vi "FTW-Container-Value-String.vi"(0 "JSON":refnum<class "FTW-Container.lvclass">, 11 "error in":errorcluster) -> (4 "JSON out":refnum<class "FTW-Container.lvclass">, 8 "Value":string, 15 "error out":errorcluster)   [LabVIEW 2015, in "FTW-Container.lvclass"]
uses:
  FTW-Container.lvclass
  FTW-Container.lvclass/FTW-Container.ctl
  <vilib>/Utility/Data Type/NI_Data Type.lvlib
panel:
  # "Inputs"
  # "Outputs"
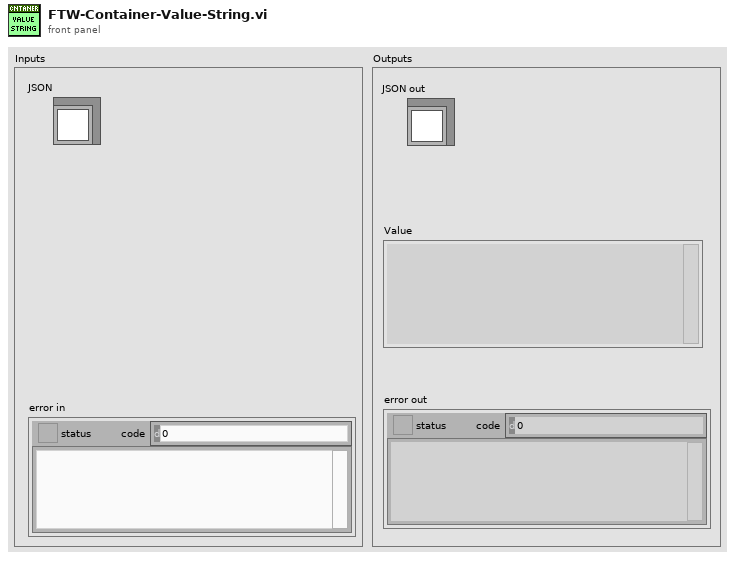
[diagram p1: front panel]
types:
  T1 = typedef "NI_Data Type.lvlib/Data Type.ctl" = enum8{"Invalid Type", "Void", "I8", "I16", "I32", "I64", "U8", "U16", "U32", "U64", "Single Float", "Double Float", "Extended Float", "Single Complex", "Double Complex", "Extended Complex", "Enum U8", "Enum U16", "Enum U32", "Enum U64", "Single Float With Unit", "Double Float With Unit", "Extended Float With Unit", "Single Complex with Unit", "Double Complex with Unit", "Extended Complex with Unit", "Boolean", "String", "Path", "Picture", "Tag", "Array", "Cluster", "Variant", "LV Variant", "Waveform", "Timestamp", "Digital Waveform", "Digital Data", "ExpressData", "Refnum", "External Data", "VI", "Poly VI", "LabVIEW Class Instance", "Fixed Point"}
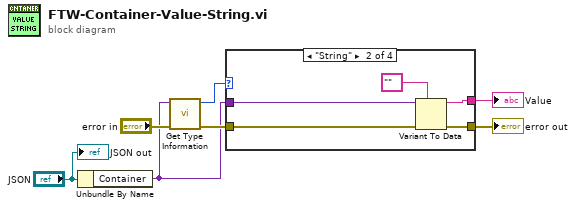
[diagram p0: block diagram]
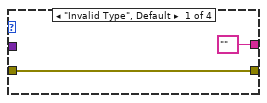
[diagram p2: hidden frame]
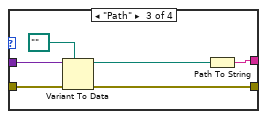
[diagram p3: hidden frame]
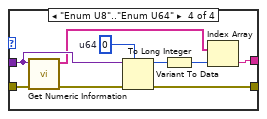
[diagram p4: hidden frame]
diagram:
  n1 = Unbundle By Name("JSON") -> ("Container"=w1:variant)
  n2 = call <vilib>:"Get Type Information.vi"("error in (no error)"="error in", "Variant"=w1) -> ("error out"=w4:errorcluster, "Type"=w3:T1)  [unwired: 5 in, 3 out]
  n3 = case shown="\"String\"" w3 {
    tunnel: w4 -> [w8 w13 w19 w28]
    tunnel: w1 -> [_ w12 w18 w25]
    tunnel: [w8 w11 w17 w27] -> w6
    tunnel: ["" ("empty string") w10 w15 w22] -> w5
    frame "Invalid Type", Default {
    }
    frame "String" {
      n4 = Variant To Data(error in=w13, type="", Variant=w12) -> (data=w10:string, error out=w11:errorcluster)
    }
    frame "Path" {
      n5 = Variant To Data(error in=w19, type=path "", Variant=w18) -> (data=w16:path, error out=w17:errorcluster)
      n6 = Path To String(path=w16) -> (string=w15:string)
    }
    frame "Enum U8".."Enum U64" {
      w29 = u64 0  # u64
      n7 = call <vilib>:"Get Numeric Information.vi"("error in (no error)"=w28, "Variant"=w25) -> ("error out"=w26:errorcluster, "Enum Names"=w24:string[])  [unwired: 6 in, 2 out]
      n8 = Variant To Data(error in=w26, type=w29, Variant=w25) -> (data=w23:u64, error out=w27:errorcluster)
      n9 = To Long Integer(number=w23) -> (32bit integer=w21:i32)
      n10 = Index Array(array=w24, index=w21) -> (element=w22:string)
    }
  }
  "error out" <- w6
  "Value" <- w5
  "JSON out" <- "JSON"
